vi "Get Name.vi"(8 "error in (no error)":errorcluster, 11 "Channel Config in":refnum<class "Channel Config.lvclass">) -> (0 "error out":errorcluster, 2 "Name":string, 3 "Channel Config out":refnum<class "Channel Config.lvclass">)   [LabVIEW 2020, in "Vecto.lvlib" / "Channel Config.lvclass"]
uses:
  Channel Config.lvclass
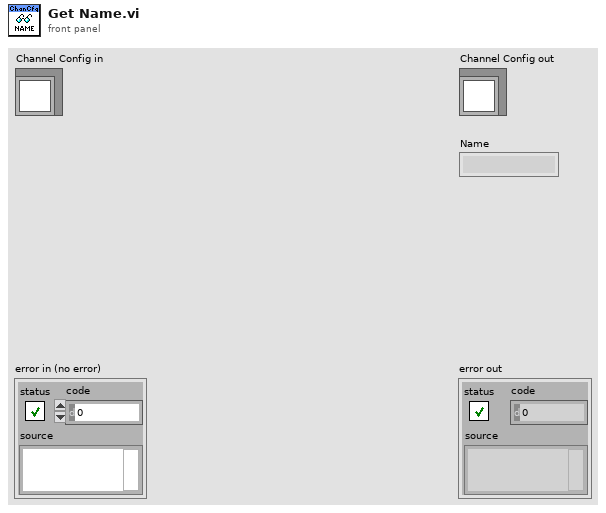
[diagram p1: front panel]
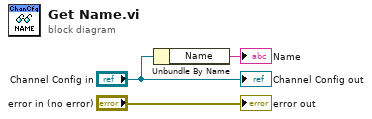
[diagram p0: block diagram]
diagram:
  n1 = Unbundle By Name("Channel Config in") -> ("Name"=→"Name":string)
  "error out" <- "error in (no error)"
  "Channel Config out" <- "Channel Config in"
